vi "ConfigStdWfrm.vi"(8 "error in (no error)":errorcluster, 11 "ClassIn":refnum<class "Keysight335XX.lvclass">) -> (0 "error out":errorcluster, 3 "ClassOut":refnum<class "Keysight335XX.lvclass">)   [LabVIEW 2014, in "FGenPlugins.lvlib" / "Keysight335XX.lvclass"]
uses:
  Keysight335XX.lvclass
  <instrlib>/Agilent 3352X Series/Agilent 3352X Series.lvlib
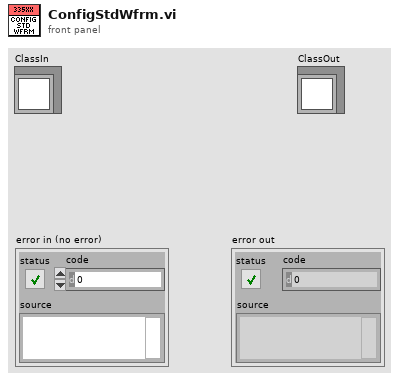
[diagram p1: front panel]
types:
  T1 = typedef "FGenPlugins.lvlib/NISTFGenPluginsBase.lvclass/StdWaveformParams.ctl" = cluster{"eWaveform":u16, "dAmplitude":dbl, "dDcOffset":dbl, "dFrequency":dbl, "dStartPhase":dbl, "dSampleRate":dbl, "dNumSamples":dbl}
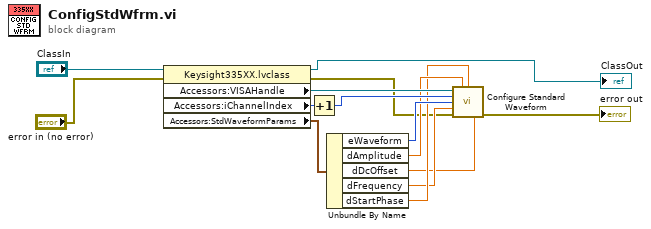
[diagram p0: block diagram]
diagram:
  n1 = property class="Keysight335XX.lvclass"(reference="ClassIn", error in="error in (no error)") -> (reference out=→"ClassOut":refnum<class "Keysight335XX.lvclass">, error out=w4:errorcluster, "Accessors:VISAHandle"=w12:refnum<visa-resource-name>, "Accessors:iChannelIndex"=w9:i32, "Accessors:StdWaveformParams"=w13:T1)
  n2 = Increment(x=w9) -> (x+1=w10:i32)
  n3 = Unbundle By Name(w13) -> ("eWaveform"=w8:u16, "dAmplitude"=w7:dbl, "dDcOffset"=w3:dbl, "dFrequency"=w5:dbl, "dStartPhase"=w6:dbl)
  n4 = call <instrlib>:"Configure Standard Waveform.vi"("VISA resource name"=w12, "Amplitude (0.1 Vpp)"=w7, "Phase Angle (0 Degree)"=w6, "Channel (1: 1)"=w10, "Waveform Function (0: Sine)"=w8, "Frequency/Sample Rate/Bandwidth (1000 Hz)"=w5, "error in (no error)"=w4, "DC Offset (0 V)"=w3) -> ("error out"=→"error out":errorcluster)  [unwired: 2 in, 5 out]
